vi "Read 2 measurement Channels Osciloscope.vi"(8 "error in (no error)":errorcluster, 10 "Read 2 channels In":T2={"TEKTRONIX- READ-CHANNELS-IN"={"Channel 1 (1: Channel 1)"=1, "Channel 2 (2: Channel 2)"=2, "Measurement Type (0: Phase)"=0}, "EDU-X-1200A- READ-CHANNELS-IN"={"Timeout (10000 ms)"=10000, "Channels"=[]}} {"EDU-X-1200A- READ-CHANNELS-IN"."Channels" items=["Channel 1"=0, "Channel 2"=1, "Channel 3"=2, "Channel 4"=3, "Waveform Memory 1"=5, "Waveform Memory 2"=6, "Serial Bus 1"=7, "Serial Bus 2"=8, "Digital Bus Low"=9, "Digital Bus High "=10, "Digital Bus 1"=11, "Digital Bus 2"=12, "External"=29, "Function 1"=32, "Function 2"=33, "Function 3"=34, "Function 4"=35, "Math 1"=36, "Math 2"=37, "Math 3"=38, "Math 4"=39, "FFT"=40, "Analog Bus"=41]; "TEKTRONIX- READ-CHANNELS-IN"."Measurement Type (0: Phase)" items=["Phase", "Delay", "DelayRR", "DelayRF", "DelayFR", "DelayFF"]; "TEKTRONIX- READ-CHANNELS-IN"."Channel 2 (2: Channel 2)" items=["Channel 1"=1, "Channel 2"=2, "Channel 3"=3, "Channel 4"=4]; "TEKTRONIX- READ-CHANNELS-IN"."Channel 1 (1: Channel 1)" items=["Channel 1"=1, "Channel 2"=2, "Channel 3"=3, "Channel 4"=4]}, 11 "Tektronicks in":refnum<class "Tektronicks.lvclass">) -> (0 "error out":errorcluster, 2 "Read 2 channels Out":T1, 3 "Tektronicks out":refnum<class "Tektronicks.lvclass">)   [LabVIEW 2020, in "Tektronicks.lvclass"]
uses:
  Tektronicks.lvclass
  TypeDefs/Read2channelsIn--cluster.ctl
  TypeDefs/Read2ChannlesOut.ctl
  Tektronicks.lvclass/Tektronicks.ctl
  <instrlib>/Tektronix TDS 200 1000 2000 Series/Tektronix TDS 200 1000 2000 Series.lvlib
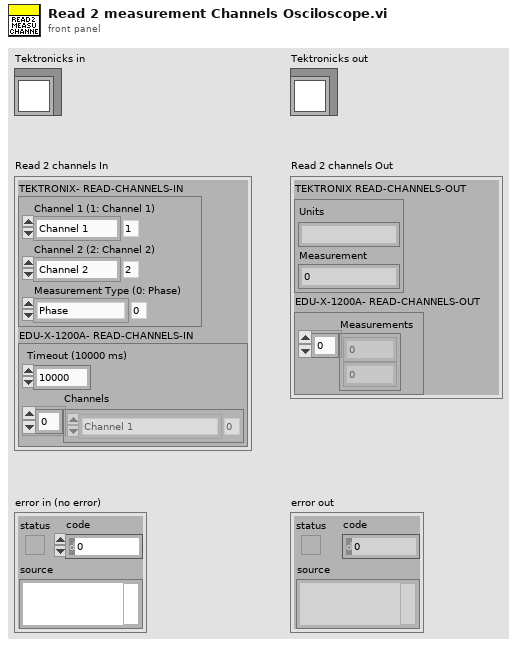
[diagram p1: front panel]
types:
  T1 = typedef "Read2ChannlesOut.ctl" = cluster{"TEKTRONIX READ-CHANNELS-OUT ":cluster{"Units":string, "Measurement":dbl}, "EDU-X-1200A- READ-CHANNELS-OUT":cluster{"Measurements":dbl[]}}
  T2 = typedef "Read2channelsIn--cluster.ctl" = cluster{"TEKTRONIX- READ-CHANNELS-IN":cluster{"Channel 1 (1: Channel 1)":i32, "Channel 2 (2: Channel 2)":i32, "Measurement Type (0: Phase)":i32}, "EDU-X-1200A- READ-CHANNELS-IN":cluster{"Timeout (10000 ms)":u32, "Channels":i32[]}}
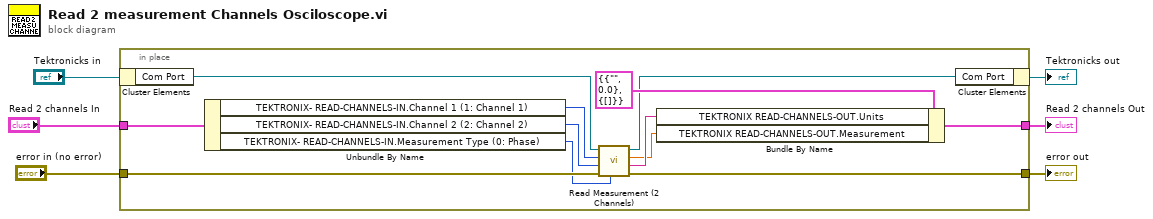
[diagram p0: block diagram]
diagram:
  n1 = in-place {
    in-place-border: "error in (no error)" -> [w18]
    in-place-border: [w17] -> w3
    in-place-border: "Read 2 channels In" -> [w16]
    in-place-border: [w12] -> w1
    n2 = in-place-cluster #1("Tektronicks in") -> ("Com Port"=w7:refnum<visa-resource-name>)
    n3 = Unbundle By Name(w16) -> ("TEKTRONIX- READ-CHANNELS-IN.Channel 1 (1: Channel 1)"=w15:i32, "TEKTRONIX- READ-CHANNELS-IN.Channel 2 (2: Channel 2)"=w14:i32, "TEKTRONIX- READ-CHANNELS-IN.Measurement Type (0: Phase)"=w13:i32)
    n4 = call <instrlib>:"Read Measurement (2 Channels).vi"("Measurement Type (0: Phase)"=w13, "error in (no error)"=w18, "Channel 2 (2: Channel 2)"=w14, "Channel 1 (1: Channel 1)"=w15, "VISA resource name"=w7) -> ("error out"=w17:errorcluster, "Units"=w10:string, "Measurement"=w9:dbl, "VISA resource name out"=w8:refnum<visa-resource-name>)  [unwired: 3 in]
    n5 = Bundle By Name(cluster=T1 {"TEKTRONIX READ-CHANNELS-OUT "={"Units"="", "Measurement"=0.0}, "EDU-X-1200A- READ-CHANNELS-OUT"={"Measurements"=[]}} ("Read 2 channels Out"), "TEKTRONIX READ-CHANNELS-OUT.Units"=w10, "TEKTRONIX READ-CHANNELS-OUT.Measurement"=w9) -> (w12:T1)
    n6 = in-place-cluster #1("Com Port"=w8) -> (→"Tektronicks out":refnum<class "Tektronicks.lvclass">)
  }
  "error out" <- w3
  "Read 2 channels Out" <- w1
